vi "Exit LabVIEW.vi"(8 "Data Flow Dependency":variant) -> ()   [LabVIEW 2021, in "Utility.lvlib"]
uses:
  Utility.lvlib
  <userlib>/_OpenG.lib/appcontrol/appcontrol.llb/openg_application_control.lvlib
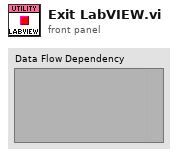
[diagram p1: front panel]
types:
  T1 = enum32{"invalid app kind", "Development System", "Run Time System", "Student Edition", "Embedded LabVIEW", "Evaluation", "Custom"}
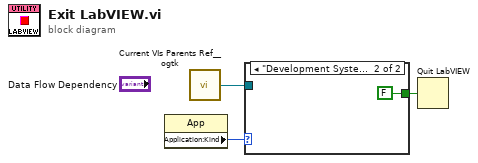
[diagram p0: block diagram]
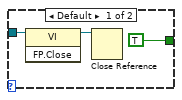
[diagram p2: hidden frame]
diagram:
  n1 = property class="App"() -> ("Application:Kind"=w1:T1)  [unwired: 2 in, 2 out]
  n2 = call <userlib>:"Current VIs Parents Ref__ogtk.vi"() -> ("Calling VI's Reference"=w2:refnum<vi>)  [unwired: 2 in]
  n3 = case shown="\"Development System\", \"Evaluation\"" w1 {
    tunnel: w2 -> [w5 _]
    tunnel: [TRUE FALSE] -> w3
    frame Default {
      n4 = invoke class="VI" method="FP.Close"(reference=w5) -> (reference out=w6:refnum<vi>)  [unwired: 2 in, 2 out]
      n5 = Close Reference(reference=w6) -> ()  [unwired: 1 in, 1 out]
    }
    frame "Development System", "Evaluation" {
    }
  }
  n6 = Quit LabVIEW(quit? (T)=w3) -> ()
